vi "Set Routing Channel Error.vi"(6 "Validation Information in":T1, 8 "error in (no error)":errorcluster, 9 "Routing Channel Error Information":T2, 11 "Routing Channel Ref in":T3 format="%.0x") -> (0 "error out":errorcluster, 1 "VeriStand Error out":errorcluster, 3 "Routing Channel Ref out":T3 format="%.0x", 4 "Validation Information out":T1)   [LabVIEW 2017, in "Routing and Faulting Scripting.lvlib"]
uses:
  Routing and Faulting Scripting.lvlib
  <vilib>/NI Veristand/Custom Device API/Custom Device Item Ref.ctl
  Routing Channel Error Information.ctl
  Validation/Validation Information.ctl
  <vilib>/NI Veristand/Custom Device API/Custom Device API.lvlib
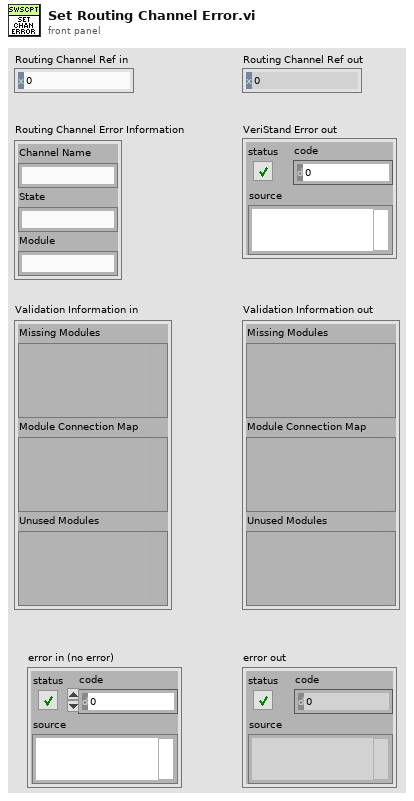
[diagram p1: front panel]
types:
  T1 = typedef "Routing and Faulting Scripting.lvlib/Validation Information.ctl" = cluster{"Missing Modules":variant, "Module Connection Map":variant, "Unused Modules":variant}
  T2 = typedef "Routing and Faulting Scripting.lvlib/Routing Channel Error Information.ctl" = cluster{"Channel Name":string, "State":string, "Module":string}
  T3 = typedef "Custom Device API.lvlib/Custom Device Item Ref.ctl" = u64
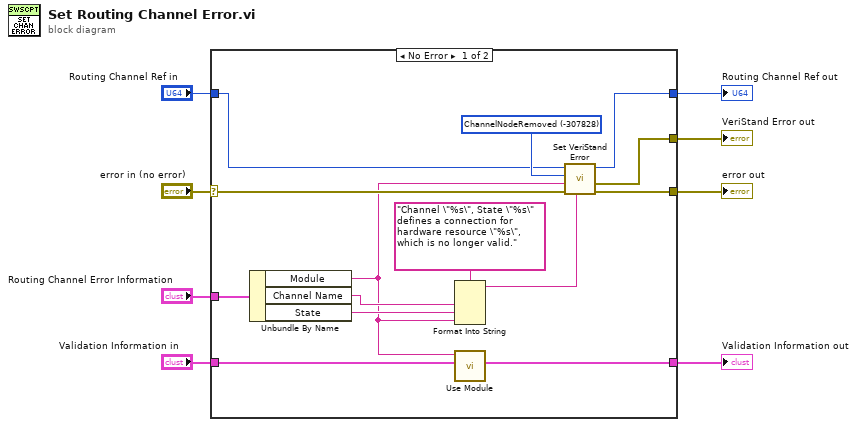
[diagram p0: block diagram]
diagram:
  n1 = case shown="No Error" "error in (no error)" {
    selector: "error in (no error)" -> [w12 w25]
    tunnel: "Routing Channel Ref in" -> [w19 w24]
    tunnel: [w18 w24] -> w7
    tunnel: "Routing Channel Error Information" -> [w17 _]
    tunnel: [w14 w25] -> w5
    tunnel: [w13 _] -> w4
    tunnel: "Validation Information in" -> [w11 w23]
    tunnel: [w10 w23] -> w1
    frame No Error {
      w21 = -307828 items=["Success"=0, "NoProjectOpen"=-307992, "SequenceCompileError"=-307988, "SessionAlreadyDeployed"=-307984, "SessionNotDeployed"=-307982, "SequenceNotFoundInSession"=-307981, "StimulusProfileSessionLocked"=-307980, "EmptyNodeName"=-307930, "NodeAlreadyExistsByName"=-307926, "NumberOfCoefficientsOutOfRange"=-307884, "DownloadFileError"=-307872, "IncorrectLogFileName"=-307871, "LogTriggerConditionSyntaxError"=-307868, "DuplicateLogSessionName"=-307867, "LogSessionNotFound"=-307865, "ChannelLengthMismatch"=-307830, "NodeNotFoundDuringCompile"=-307829, "ChannelNodeRemoved"=-307828, "NotAChannel"=-307825, "NotAWaveform"=-307824, "STIFileError"=-307784, "DependenciesCycle"=-307783, "ChannelNotFoundInLogFile"=-307782, "ChannelGroupNotFoundInLogFile"=-307781, "GatewayNotOnLocalhost"=-307780, "NotEnoughDynamicDataSharingSpace"=-307738, "TargetMissingDataSharingDevice"=-307737, "ChannelMappingsSizeMismatch"=-307728, "DuplicateChannelAliasMappings"=-307711, "NotAnInlineCustomDevice"=-307710, "IncompatibleModel"=-307703, "ModelDimensionMismatch"=-307702, "SLSCChassisLoadFailed"=-307691, "TargetDisabled"=-307689, "MismatchedLengths"=-307687, "TargetInvalid"=-307686, "ParameterNotFound"=-307685, "ServerPortAlreadyInUse"=-307684, "TargetDisconnected"=-307682, "ServiceConfigurationFile"=-307681, "ModelParameterFileParseError"=-307680, "NoActionRequired"=-307677, "InputParameterInvalid"=-307676, "HostRunningDifferentSystemDefinition"=-307671, "ChannelNotScalable"=-307668, "ChannelCannotBeFaulted"=-307666, "ChannelNotWritable"=-307665, "ChannelNotReadable"=-307664, "Timeout"=-307663, "NodeNotFound"=-307662, "SystemDefinitionDeploymentFailure"=-307661, "SystemDefinitionDeploymentTimeout"=-307660, "EmptyPassword"=-307659, "SystemDefinitionAlreadyActive"=-307658, "InvalidConfigurationPassword"=-307657, "NoSystemDefinitionLoaded"=-307656, "ComponentNotAvailable"=-307655, "NotDeployed"=-307654, "InvalidFile"=-307653, "FailedServerConnection"=-307652, "FunctionNotSupported"=-307651, "UnexpectedError"=-307650, "UnmappedAlias"=-307617, "InvalidStreamConditionForDataType"=-307554, "WaveformDataTypeMismatch"=-307553, "InvalidDaqPluginFile"=-307526, "FileVersionUnsupported"=-307525] ("NationalInstruments.VeriStand.ErrorCode")
      n2 = Unbundle By Name(w17) -> ("Module"=w9:string, "Channel Name"=w16:string, "State"=w15:string)
      n3 = Format Into String(format string="Channel \"%s\", State \"%s\" defines a connection for hardware resource \"%s\", which is no longer valid.", w16, w15, w9) -> (resulting string=w20:string)  [unwired: 2 in, 1 out]
      n4 = call "Use Module.vi"("Validation Information in"=w11, "Module Path"=w9) -> ("Validation Information out"=w10:T1)  [unwired: 8 in, 1 out]
      n5 = call "Set VeriStand Error.vi"("message"=w20, "error in (no error)"=w12, "key"=w9, "errCode"=w21, "Custom Device Item Ref in"=w19) -> ("error out"=w14:errorcluster, "VeriStand Error out"=w13:errorcluster, "Custom Device Item Ref out"=w18:T3)  [unwired: 4 in]
    }
    frame Error {
    }
  }
  "Routing Channel Ref out" <- w7
  "error out" <- w5
  "VeriStand Error out" <- w4
  "Validation Information out" <- w1
